vi "Shift coordinates (IMAQ to SLM).vi"(5 "Trap cluster":T1, 7 "Coordinate mapping \n(IMAQ to SLM)":T2) -> (0 "X (SLM)":sgl[](array[numeric]), 1 "Y (SLM)":sgl[](array[numeric]), 2 "Intensities":sgl[](array[numeric]), 3 "Number of traps":i32, 4 "Z (SLM)":sgl[](array[numeric]))   [LabVIEW 2011]
uses:
  Trap cluster.ctl
panel:
  out "element":T1
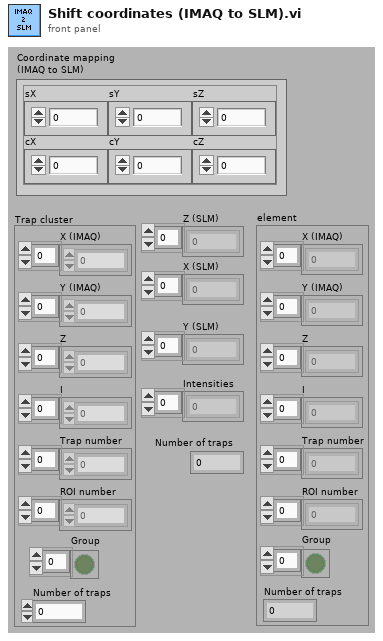
[diagram p1: front panel]
types:
  T1 = typedef "Trap cluster.ctl" = cluster{"X (IMAQ)":sgl[], "Y (IMAQ)":sgl[], "Z":sgl[], "I":sgl[], "Trap number":i32[], "ROI number":i32[], "Number of traps":i32, "Group":bool[]}
  T2 = cluster{"cZ":sgl, "cY":sgl, "cX":sgl, "sZ":sgl, "sY":sgl, "sX":sgl}
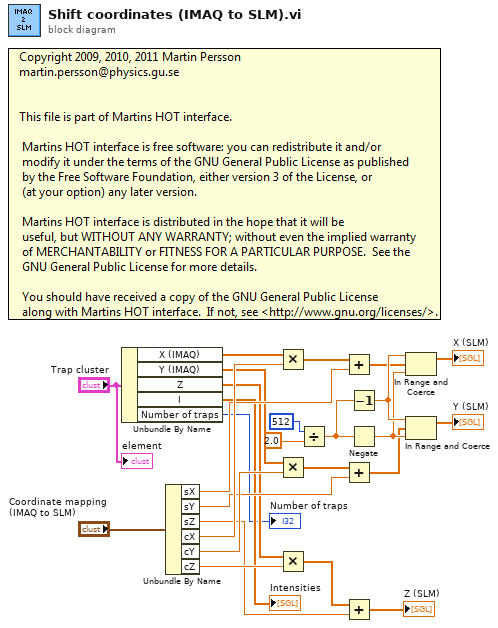
[diagram p0: block diagram]
diagram:
  n1 = Unbundle By Name("Trap cluster") -> ("X (IMAQ)"=w14:sgl[], "Y (IMAQ)"=w13:sgl[], "Z"=w12:sgl[], "I"=→"Intensities":sgl[], "Number of traps"=→"Number of traps":i32)
  n2 = Unbundle By Name("Coordinate mapping \n(IMAQ to SLM)") -> ("sX"=w21:sgl, "sY"=w22:sgl, "sZ"=w23:sgl, "cX"=w24:sgl, "cY"=w25:sgl, "cZ"=w26:sgl)
  n3 = Multiply(x=w14, y=w24) -> (x*y=w18:sgl[])
  n4 = Multiply(x=w13, y=w25) -> (x*y=w19:sgl[])
  n5 = Multiply(x=w12, y=w26) -> (x*y=w20:sgl[])
  n6 = Divide(x=512 ("SLM size"), y=sgl 2.0) -> (x/y=w9:sgl)
  n7 = Add(x=w18, y=w21) -> (x+y=w7:sgl[])
  n8 = Add(x=w19, y=w22) -> (x+y=w6:sgl[])
  n9 = Add(x=w20, y=w23) -> (x+y=→"Z (SLM)":sgl[])
  n10 = Decrement(x=w9) -> (x-1=w10:sgl)
  n11 = Negate(x=w9) -> (-x=w8:sgl)
  n12 = In Range and Coerce(upper limit=w10, x=w7, lower limit=w8) -> (coerced(x)=→"X (SLM)":sgl[])  [unwired: 1 out]
  n13 = In Range and Coerce(upper limit=w10, x=w6, lower limit=w8) -> (coerced(x)=→"Y (SLM)":sgl[])  [unwired: 1 out]
  "element" <- "Trap cluster"
